vi "ArrayDevScanPar.vi"(6 "CurPointInd":i32, 7 "VarParams":string[][](array[string]), 8 "error in":errorcluster caption="entrée d'erreur (pas d'erreur)", 9 "IndCourbe":i64, 10 "DevID":i32, 11 "Experiment.lvclass In":refnum<class "Experiment.lvclass">) -> (0 "error out":errorcluster caption="sortie d'erreur", 1 "ReuseVarPar":bool, 2 "ScanPar":T1={"Entête"="", "Scan list"=[], "NbCourbe"=1, "IndCourbe"=0, "NomDon"=["RTêta;", "X&Y;"], "Session "=0, "Date"="", "Time"="", "VarParams"=[], "UserName"="", "ScanTableSize"=[], "VarPar list"=[], "DescKeyword"=""} caption="ScanParams", 3 "FileNmDTString":string, 4 "SaveArrDat":bool)   [LabVIEW 2019, in "Experiment.lvclass"]
uses:
  Experiment.lvclass
  Interface Class/ScanParams.ctl
  Experiment.lvclass/Experiment.ctl
  DevicesClass/BaseDevice/BaseDevice.lvclass
  Interface Class/Interface.lvclass
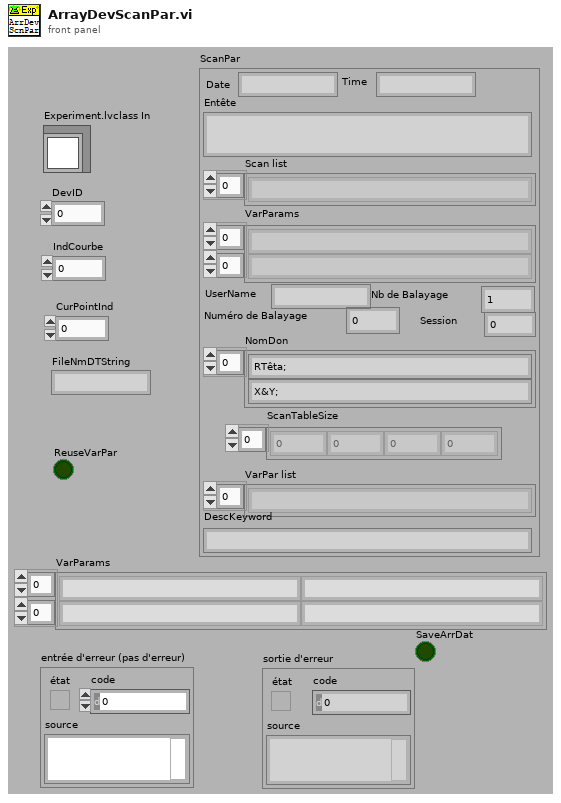
[diagram p1: front panel]
types:
  T1 = typedef "Interface.lvclass/ScanParams.ctl" = cluster{"Entête":string, "Scan list":string[], "NbCourbe":i32, "IndCourbe":i64, "NomDon":string[], "Session ":i32, "Date":string, "Time":string, "VarParams":string[][], "UserName":string, "ScanTableSize":i32[], "VarPar list":string[], "DescKeyword":string}
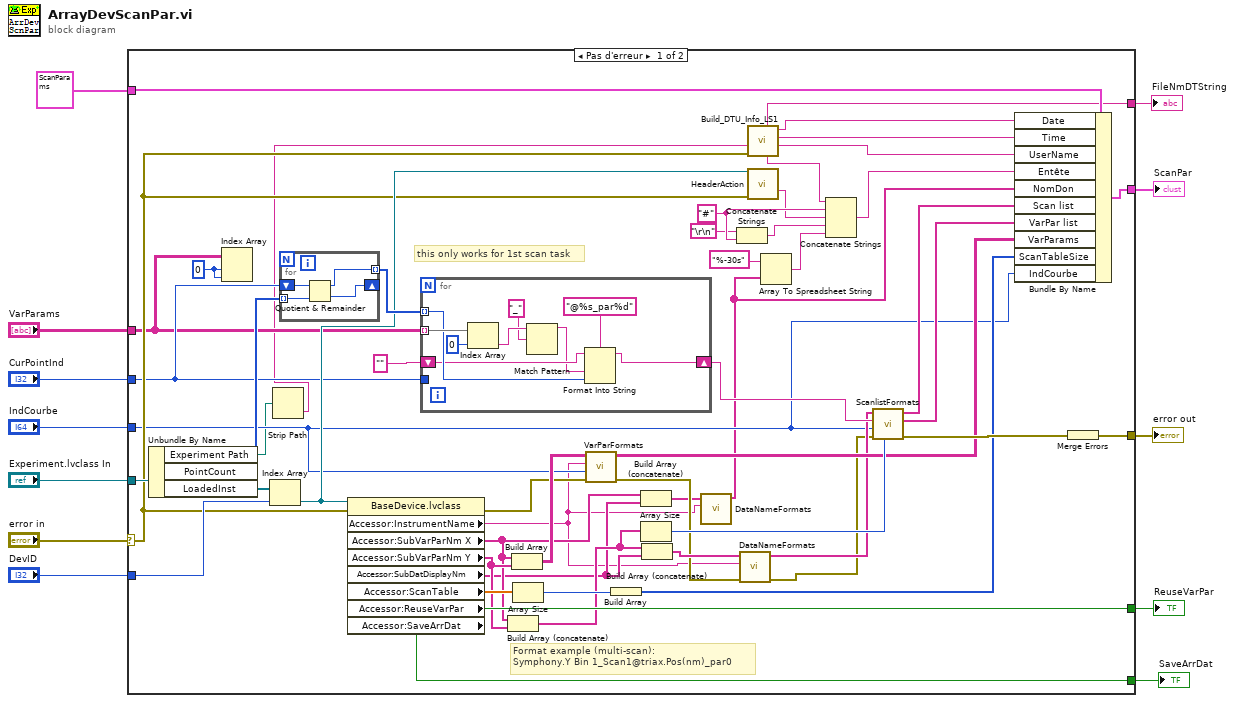
[diagram p0: block diagram]
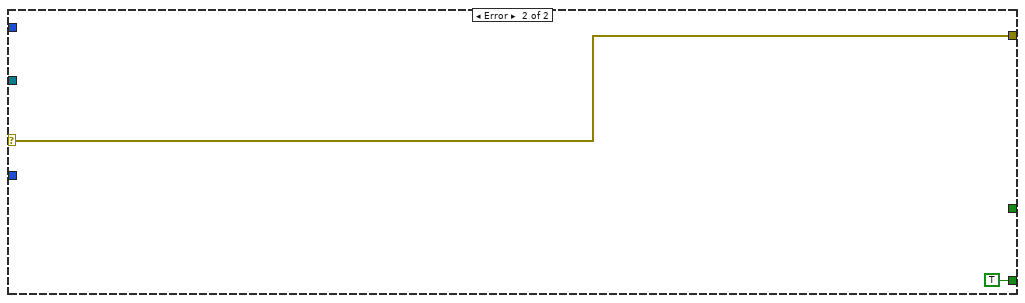
[diagram p2: hidden frame]
diagram:
  n1 = case shown="Pas d'erreur" "error in" {
    selector: "error in" -> [w46 w80]
    tunnel: [w65 w80] -> w11
    tunnel: "Experiment.lvclass In" -> [w62 _]
    tunnel: "IndCourbe" -> [w21 _]
    tunnel: "DevID" -> [w64 _]
    tunnel: "CurPointInd" -> [w45 _]
    tunnel: "VarParams" -> [w44 _]
    tunnel: T1 {"Entête"="", "Scan list"=[], "NbCourbe"=1, "IndCourbe"=0, "NomDon"=["RTêta;", "X&Y;"], "Session "=0, "Date"="", "Time"="", "VarParams"=[], "UserName"="", "ScanTableSize"=[], "VarPar list"=[], "DescKeyword"=""} ("ScanParams") -> [w55 _]
    tunnel: [w42 _] -> w4
    tunnel: [w33 _] -> w3
    tunnel: [w32 _] -> w2
    tunnel: [w15 TRUE ("Accessor:SaveArrDat")] -> w1
    frame No Error {
      w43 = 0 ("indice (ligne)")
      w60 = "#" ("chaîne")
      # "this only works for 1st scan task"
      # "Format example (multi-scan):\nSymphony.Y Bin 1_Scan1@triax.Pos(nm)_par0"
      n2 = Unbundle By Name(w62) -> ("Experiment Path"=w14:path, "PointCount"=w58:i32[], "LoadedInst"=w63:refnum<class "BaseDevice.lvclass">[])
      n3 = Index Array(array=w44, index (row)=w43, index (col)=w43) -> ()  [unwired: 1 out]
      n4 = Index Array(array=w63, index=w64) -> (element=w56:refnum<class "BaseDevice.lvclass">)
      n5 = Strip Path(path=w14) -> (name=w13:string)  [unwired: 1 out]
      n6 = for {
        tunnel: w58 -> [w68] mode=indexing
        shift-right: [w67] -> _
        shift-left: w45 -> [w69]
        tunnel: [w66] -> w57 mode=indexing
        n7 = Quotient & Remainder(x=w69, y=w68) -> (x-y*floor(x/y)=w66:i32, floor(x/y)=w67:i32)
      }
      n8 = property class="BaseDevice.lvclass"(reference=w56, error in=w46) -> (error out=w37:errorcluster, "Accessor:InstrumentName"=w17:string, "Accessor:SubVarParNm X"=w27:string[], "Accessor:SubVarParNm Y"=w29:string[], "Accessor:SubDatDisplayNm"=w26:string[], "Accessor:ScanTable"=w34:dbl[], "Accessor:ReuseVarPar"=w32:bool, "Accessor:SaveArrDat"=w15:bool)  [unwired: 1 out]
      n9 = for {
        tunnel: w44 -> [w78] mode=indexing
        tunnel: w45 -> [_]
        shift-right: [w75] -> w38
        shift-left: "" -> [w73]
        tunnel: w57 -> [w74] mode=indexing
        n10 = Index Array(array=w78, index=0 ("indice")) -> (element=w72:string)
        n11 = Match Pattern(string=w72, regular expression="_" ("expression régulière")) -> (before substring=w71:string)  [unwired: 1 in, 3 out]
        n12 = Format Into String(format string="@%s_par%d" ("chaîne de format"), initial string=w73, w71, w74) -> (resulting string=w75:string)  [unwired: 1 in, 1 out]
      }
      n13 = Build Array (concatenate)(w27, w29) -> (w28:string[])
      n14 = Build Array(w27, w29) -> (w41:string[][])
      n15 = Array Size(array=w34) -> (size(s)=w47:i32)
      n16 = call "VarParFormats.vi"("ErrorIn(No Error)"=w37, "IndCourbe"=w21, "InstrumentName"=w17, "VarParArr"=w41) -> ("Err Out"=w23:errorcluster, "VarParArrOut"=w30:string[][])  [unwired: 6 in]
      n17 = Build Array(w47) -> (w31:i32[])
      n18 = Build Array (concatenate)(w27, w26) -> (w18:string[])
      n19 = Array Size(array=w28) -> (size(s)=w36:i32)
      n20 = Build Array (concatenate)(w28, w26) -> (w25:string[])
      n21 = call "DataNameFormats.vi"("InstrumentName"=w17, "DataNameArr"=w18) -> ("DataNameArrOut"=w16:string[])  [unwired: 8 in, 1 out]
      n22 = Concatenate Strings("\r\n", w60) -> (w20:string)
      n23 = call "DataNameFormats.vi"("ErrorIn(No Error)"=w23, "InstrumentName"=w17, "DataNameArr"=w25) -> ("Err Out"=w22:errorcluster, "DataNameArrOut"=w24:string[])  [unwired: 7 in]
      n24 = call "Build_DTU_Info_LS1.vi"("error in"=w46, "Experiment Path"=w13) -> ("ScanParUser"=w50:string, "ScanParTime"=w51:string, "ScanParDate"=w54:string, "DTU_HdrStr"=w52:string, "FileNmDTString"=w33:string)  [unwired: 3 in, 2 out]
      n25 = call-dynamic "HeaderAction.vi"("Device en entrée"=w56, "error in (no error)"=w46) -> ("HeaderString"=w53:string)  [unwired: 7 in, 6 out]
      n26 = Array To Spreadsheet String(array=w16, 3:"%-30s" ("format string")) -> (spreadsheet string=w48:string)  [unwired: 1 in]
      n27 = Concatenate Strings(w52, w60, w53, w20, w48) -> (w49:string)
      n28 = call "ScanlistFormats.vi"("FirstMeasNmInd"=w36, "ErrorIn(No Error)"=w22, "IndCourbe"=w21, "DatNmSuffix"=w38, "DatNmArr"=w24) -> ("Err Out"=w35:errorcluster, "VarParList"=w39:string[], "ScanList"=w40:string[])  [unwired: 4 in]
      n29 = Bundle By Name(cluster=w55, "Date"=w54, "Time"=w51, "UserName"=w50, "Entête"=w49, "NomDon"=w16, "Scan list"=w40, "VarPar list"=w39, "VarParams"=w30, "ScanTableSize"=w31, "IndCourbe"=w21) -> (w42:T1)
      n30 = Merge Errors(w35) -> (w65:errorcluster)
    }
    frame Error {
    }
  }
  "error out" <- w11
  "ScanPar" <- w4
  "FileNmDTString" <- w3
  "ReuseVarPar" <- w2
  "SaveArrDat" <- w1
